vi "generate default line.vi"(8 "error in":errorcluster, 11 "objects in":T1) -> (0 "error out":errorcluster, 2 "Line":T2, 3 "objects out":T1)   [LabVIEW 2021, in "Multiplexer editor node.lvclass"]
doc: "Generates a new line with default settings."
uses:
  Multiplexer editor node.lvclass
  configuration/Line.ctl
  <vilib>/NI/Tag Bus Module Framework/channel/TBM channel.lvclass
  <vilib>/NI/DCAF/Tag Editor Core/Table API/Table Manager/object ref.ctl
  <vilib>/NI/DCAF/Tag Editor Core/Configuration Editor/Classes/Engine Parent/Engine Parent Editor Node.lvclass
  <vilib>/NI/DCAF/Tag Editor Core/Configuration Editor/Classes/Module editor node/module editor node.lvclass
  C:/Program Files (x86)/National Instruments/LabVIEW 2021/vi.lib/NI/Configuration Framework/serializable node/NISE_CEF_serializable node.lvclass
  configuration/Multiplexer configuration.lvclass
  <vilib>/NI/Configuration Framework/serializable configuration/NISE_CEF_serializable configuration.lvclass
  <vilib>/NI/DCAF/Tag Editor Core/Table API/Table Manager/Table Manager.lvclass
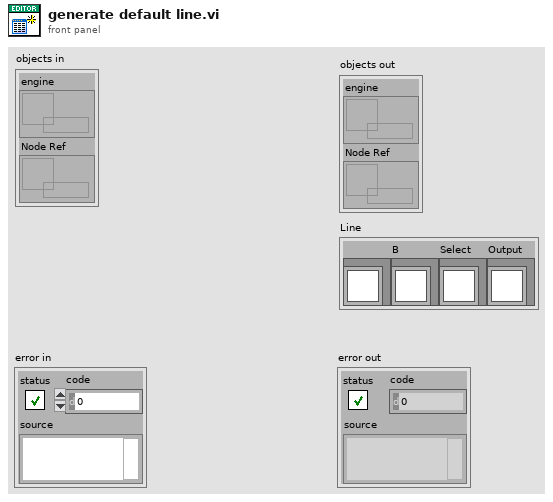
[diagram p1: front panel]
types:
  T1 = typedef "Table Manager.lvlib/Table Manager.lvclass/object ref.ctl" = cluster{"engine":refnum<data-value>, "Node Ref":refnum<data-value>}
  T2 = typedef "Multiplexer configuration.lvclass/Line.ctl" = cluster{"A":refnum<class "TBM channel.lvclass">, "B":refnum<class "TBM channel.lvclass">, "Select":refnum<class "TBM channel.lvclass">, "Output":refnum<class "TBM channel.lvclass">}
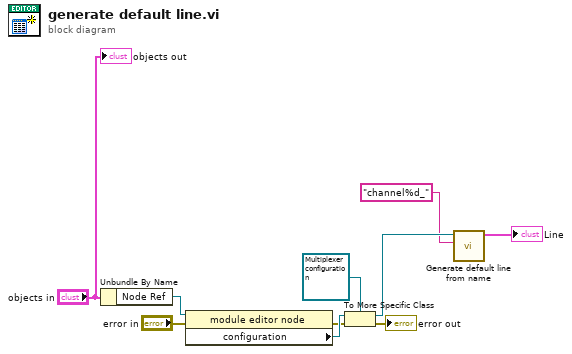
[diagram p0: block diagram]
diagram:
  n1 = Unbundle By Name("objects in") -> ("Node Ref"=w9:refnum<data-value>)
  n2 = property class="module editor node"(reference=w9, error in="error in") -> (error out=w4:errorcluster, "configuration"=w8:refnum<class "NISE_CEF_serializable configuration.lvclass">)  [unwired: 1 out]
  n3 = To More Specific Class(target class=refnum<class "Multiplexer configuration.lvclass"> refnum ("module configuration in"), reference=w8, error in=w4) -> (specific class reference=w7:refnum<class "Multiplexer configuration.lvclass">, error out=→"error out":errorcluster)
  n4 = call "Generate default line from name.vi"("Name"="channel%d_" ("format string"), "Multiplexer configuration in"=w7) -> ("Line"=→"Line":T2)  [unwired: 9 in]
  "objects out" <- "objects in"
